vi "token--image--dark.vi"() -> ()   [LabVIEW 2021]
panel:
  in  "template--token--dark":bool
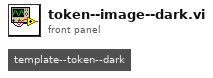
[diagram p1: front panel]
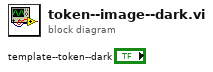
[diagram p0: block diagram]
diagram:
